vi "BinaryToMilimeter.vi"(11 "Hex string":string) -> (3 "Distance(mm)":dbl)   [LabVIEW 2024]
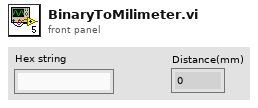
[diagram p1: front panel]
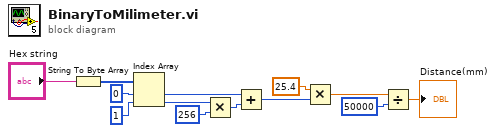
[diagram p0: block diagram]
diagram:
  n1 = String To Byte Array(string="Hex string") -> (unsigned byte array=w1:u8[])
  n2 = Index Array(array=w1, index #1=0 ("index"), index #2=1 ("index")) -> (element #1=w7:u8, element #2=w8:u8)
  n3 = Multiply(x=w8, y=u16 256) -> (x*y=w6:u16)
  n4 = Add(x=w7, y=w6) -> (x+y=w5:u16)
  n5 = Multiply(x=25.4, y=w5) -> (x*y=w4:dbl)
  n6 = Divide(x=w4, y=u32 50000) -> (x/y=→"Distance(mm)":dbl)
